vi "ShowRobotPosition.vi"() -> ()   [LabVIEW 2009, in "Host.lvlib"]
uses:
  Host.lvlib
  Draw.lvlib
  NetworkVarTarget.lvlib
panel:
  out "Image Out":T1(plugin-control)
  in  "Set goal":bool
  out "Robot Position":cluster{"X":dbl, "Y":dbl, "Angle":dbl}
  in  "Goal":cluster{"X":dbl, "Y":dbl}
  out "Map":picture
  in  "stop":bool
  in  "Reset Map":bool
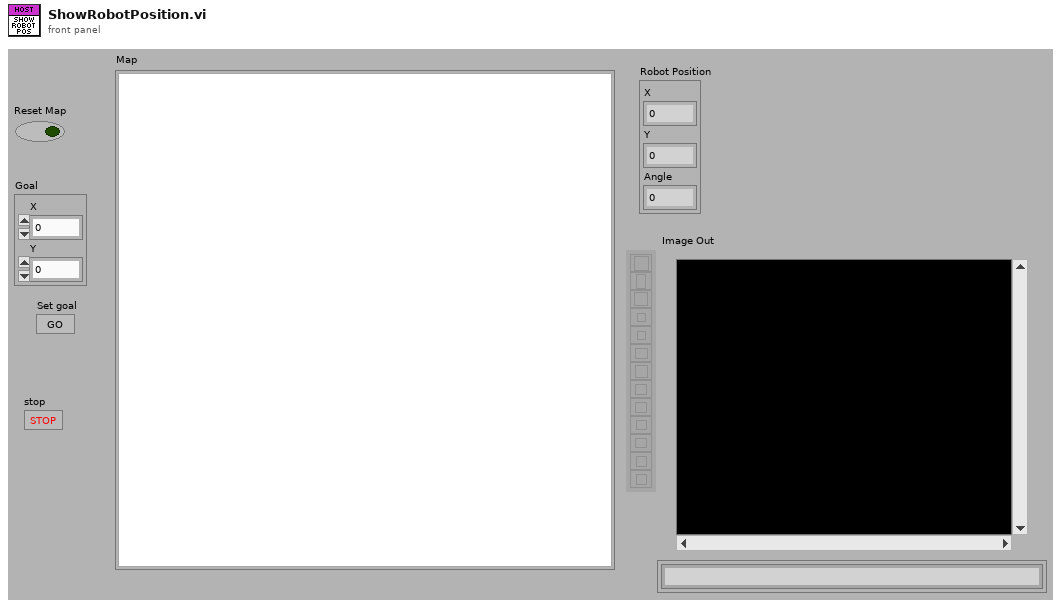
[diagram p1: front panel]
types:
  T1 = typedef "IMAQ Image.ctl" = refnum<image>
  T2 = cluster{"Width":u16, "Style":enum32{"Solid", "Dash", "Dot", "DashDot", "DashDotDot"}}
  T3 = cluster{"Position":cluster{"X":dbl, "Y":dbl, "Angle":dbl}, "Speed":cluster{"Left":dbl, "Right":dbl}}
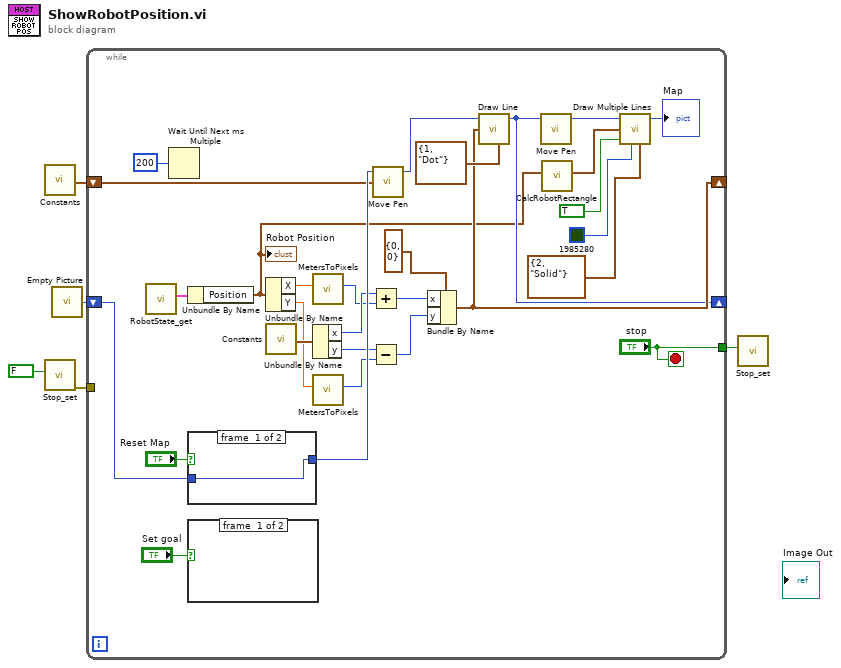
[diagram p0: block diagram]
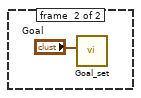
[diagram p2: hidden frame]
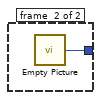
[diagram p3: hidden frame]
diagram:
  n1 = call "Constants.vi"() -> ("PictureCenterPoint"=w1:cluster{"x":i32, "y":i32})  [unwired: 16 in, 3 out]
  n2 = call "Stop_set.vi"("Stop? (F)"=FALSE ("Stop")) -> ("error out"=w4:errorcluster)  [unwired: 10 in]
  n3 = call "Empty Picture"() -> ("empty picture"=w5:picture)
  n4 = while {
    shift-right: [w24] -> _
    shift-left: w5 -> [w30]
    shift-right: [w29] -> _
    shift-left: w1 -> [w26]
    tunnel: w4 -> [_]
    tunnel: ["stop"] -> w2
    stop <- "stop" stop-if-true
    n5 = call "RobotState_get.vi"() -> ("RobotState"=w12:T3)  [unwired: 10 in, 1 out]
    n6 = Wait Until Next ms Multiple(millisecond multiple=u32 200) -> ()  [unwired: 1 out]
    n7 = Unbundle By Name(w12) -> ("Position"=w11:cluster{"X":dbl, "Y":dbl, "Angle":dbl})
    "Robot Position" <- w11
    n8 = case shown="True" "Reset Map" {
      tunnel: w30 -> [w36 _]
      tunnel: [w36 w37] -> w28
      frame #0 {
      }
      frame #1 {
        n9 = call "Empty Picture"() -> ("empty picture"=w37:picture)
      }
    }
    n10 = case shown="True" "Set goal" {
      frame #0 {
      }
      frame #1 {
        n11 = call "Goal_set.vi"("Goal"="Goal") -> ()  [unwired: 10 in, 1 out]
      }
    }
    n12 = Unbundle By Name(w11) -> ("X"=w8:dbl, "Y"=w10:dbl)
    n13 = call "Constants.vi"() -> ("PictureCenterPoint"=w13:cluster{"x":i32, "y":i32})  [unwired: 16 in, 3 out]
    n14 = call "MetersToPixels.vi"("meters"=w8) -> ("pixels"=w7:i32)  [unwired: 10 in]
    n15 = Unbundle By Name(w13) -> ("x"=w18:i32, "y"=w16:i32)
    n16 = call "MetersToPixels.vi"("meters"=w10) -> ("pixels"=w9:i32)  [unwired: 10 in]
    n17 = Add(x=w18, y=w7) -> (x+y=w17:i32)
    n18 = Subtract(x=w16, y=w9) -> (x-y=w15:i32)
    n19 = call <vilib>:"Move Pen.vi"("new position"=w26, "picture"=w28) -> ("new picture"=w27:picture)  [unwired: 3 in]
    n20 = Bundle By Name(cluster=cluster{"x":i16, "y":i16} {"x"=0, "y"=0} ("end point"), "x"=w17, "y"=w15) -> (w29:cluster{"x":i16, "y":i16})
    n21 = call <vilib>:"Draw Line.vi"("picture"=w27, "end point"=w29, "pen"=T2 {"Width"=1, "Style"=enum."Dot"}) -> ("new picture"=w24:picture)  [unwired: 6 in]
    n22 = call <vilib>:"Move Pen.vi"("picture"=w24) -> ("new picture"=w25:picture)  [unwired: 4 in]
    n23 = call "CalcRobotRectangle.vi"("Position (m and rad)"=w11) -> ("line endpoints"=w19:cluster{"x":i16, "y":i16}[])  [unwired: 10 in]
    n24 = call <vilib>:"Draw Multiple Lines.vi"("picture"=w25, "line endpoints"=w19, "fill?(F)"=TRUE, "color(black)"=u32 1985280, "pen"=T2 {"Width"=2, "Style"=enum."Solid"}) -> ("new picture"=→"Map":picture)  [unwired: 4 in]
  }
  n25 = call "Stop_set.vi"("Stop? (F)"=w2) -> ()  [unwired: 10 in, 1 out]
